vi "GeneralSettings.vi"(11 "notifier":refnum<notifier>) -> ()   [LabVIEW 2013, in "main.lvlib"]
uses:
  main.lvlib
  Controls/Enum Variables.ctl
  Controls/Enum Save Action Events.ctl
  Controls/Enum User Events.ctl
panel:
  out "JournalPositionLabel":string="Journal position i Excel" caption="generalSettingsString"
  in  "CellStr2":string="H49" caption="Højre/Nederst"
  in  "CellStr1":string="A1" caption="Venstre/Øverst"
  in  "LanguageSelectionRing":u16(ring) caption="Sprog" items=["Dansk", "English", "Français"]
  out "generalSettingsString":string
  in  "hyphenationDialogBox":bool caption="Hyphenation"
  # "Ex: A1"
  # "Ex: H49"
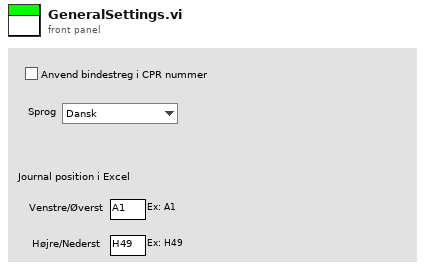
[diagram p1: front panel]
types:
  T1 = typedef "main.lvlib/Enum Variables.ctl" = enum16{"SetAcqFilter", "GetAcqFilter", "Set Filter", "Get Filter", "Set Height", "Get Height", "Set Recorded Height", "Get Recorded Height", "Set Blue Pressure", "Get Blue Pressure", "Set Red Pressure", "Get Red Pressure", "Init", "Reset Pressure", "Set Red Cursors", "Get Red Cursors", "Set Blue Cursors", "Get Blue Cursors", "Set Language", "Get Language", "Set Active Graphs", "Get ActiveGraphs", "Set Method", "Get Method", "Set Encryption", "Get Encryption", "Set ExcelVersion", "Get ExcelVersion", "Set DICOM Avail", "Get DICOM Avail", "Set DICOM Encode", "Get DICOM Encode", "Set JournalExport", "Get JournalExport", "Set Sequence", "Get Sequence", "Set DAQ Connected", "Get DAQ Connected", "Set Current Graph", "Get Current Graph", "Set General Settings", "Get Hyphenation", "Set Arm Calc Method", "Get Arm Calc Method", "Set Dicom Tags", "Get Dicom Tags", "Set BT Serial", "Get BT Serial", "Set BT Accepted Serials", "Get BT Accepted Serials", "Get BT License", "Set BT License"}
  T2 = typedef "main.lvlib/Enum Save Action Events.ctl" = enum16{"LoadReportPath", "SaveReportPath", "Load Graph Path", "Save Graph Path", "LoadDataPath", "SaveDataPath", "Load Template Path", "Save Template Path", "Load PressureFactor", "Save PressureFactor", "Init", "Load Listbox", "Save Listbox", "LoadHospInfo", "SaveHospInfo", "Load DICOM Activation", "Save DICOM Activation", "LoadDICOMInfoWL", "SaveDICOMInfoWL", "LoadDICOMInfoPACS", "SaveDICOMInfoPACS", "Load ArmCalcMethod", "Save ArmCalcMethod", "LoadItemTags", "SaveItemTags", "LoadDICOMEncoding", "SaveDICOMEncoding", "LoadJournalType", "SaveJournalType", "LoadAcqFilterType", "SaveAcqFilterType", "Load Sequence", "Save Sequence", "Load Acquisition Mode", "Save Acquisition Mode", "Load General Settings", "Save General Settings", "Load Language", "Save Language", "Load Dicom Tags", "Save Dicom Tags", "Load BT Serial", "Save BT Serial", "Load BT License", "Save BT License"}
  T3 = typedef "main.lvlib/Enum User Events.ctl" = enum16{"User Event", "Init"}
  T4 = cluster{"hyphenationDialogBox":bool, "LanguageSelectionRing":u16, "CellStr1":string, "CellStr2":string}
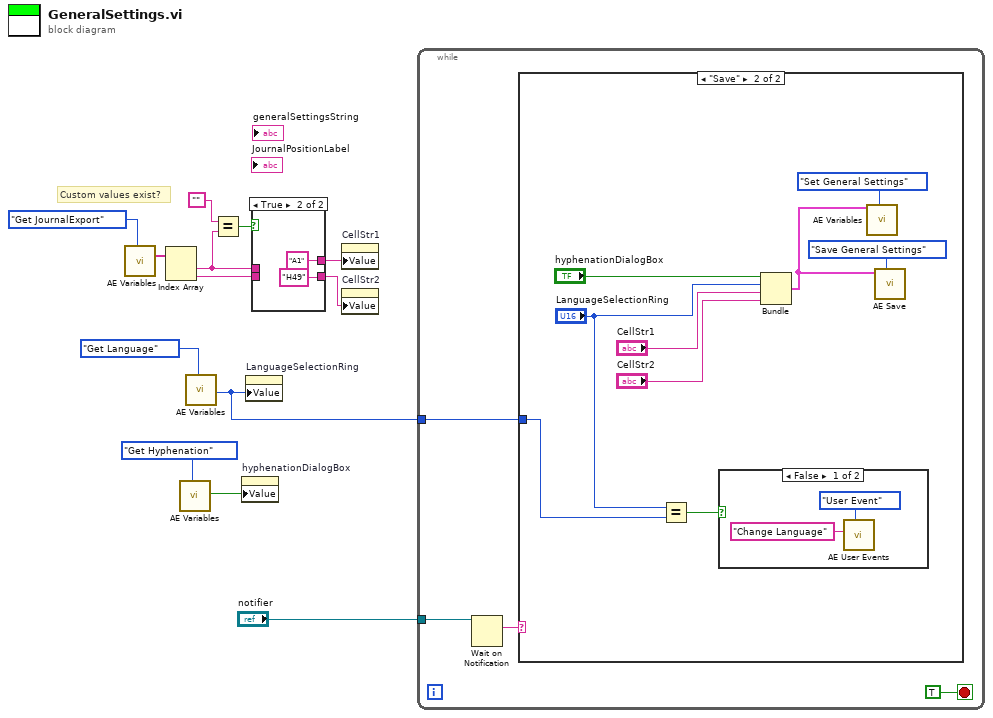
[diagram p0: block diagram]
diagram:
  # "Custom values exist?"
  n1 = call "AE Variables.vi"("Action"=Enum_Variables."Get JournalExport") -> ("stringArray"=w7:string[])  [unwired: 11 in, 7 out]
  n2 = Index Array(array=w7) -> (element #1=w4:string, element #2=w3:string)  [unwired: 2 in]
  n3 = call "AE Variables.vi"("Action"=Enum_Variables."Get Hyphenation") -> ("BooleanOut"=w11:bool)  [unwired: 11 in, 7 out]
  n4 = call "AE Variables.vi"("Action"=Enum_Variables."Get Language") -> ("RingOut"=w9:u16)  [unwired: 11 in, 7 out]
  n5 = Equal?(x="", y=w4) -> (x = y?=w5:bool)
  n6 = property on="hyphenationDialogBox" class="Bool (strict)"("Value"=w11) -> ()  [unwired: 2 in, 2 out]
  n7 = property on="LanguageSelectionRing" class="Ring (strict)"("Value"=w9) -> ()  [unwired: 2 in, 2 out]
  n8 = case shown="True" w5 {
    tunnel: w4 -> [w15 _]
    tunnel: w3 -> [w14 _]
    tunnel: [w15 "A1"] -> w2
    tunnel: [w14 "H49"] -> w1
    frame False {
    }
    frame True {
    }
  }
  n9 = property on="CellStr1" class="Str"("Value"=w2) -> ()  [unwired: 2 in, 2 out]
  n10 = property on="CellStr2" class="Str"("Value"=w1) -> ()  [unwired: 2 in, 2 out]
  n11 = while {
    tunnel: "notifier" -> [w20]
    tunnel: w9 -> [w18]
    stop <- TRUE stop-if-true
    n12 = Wait on Notification(notifier=w20) -> (notification=w21:string)  [unwired: 3 in, 3 out]
    n13 = case shown="\"Save\"" w21 {
      tunnel: w18 -> [_ w26]
      frame "Cancel", Default {
      }
      frame "Save" {
        n14 = Equal?(x="LanguageSelectionRing", y=w26) -> (x = y?=w25:bool)
        n15 = case shown="False" w25 {
          frame False {
            n16 = call "AE User Events.vi"("Action"=Enum_User_Events."User Event", "User Event"="Change Language") -> ()  [unwired: 8 in, 2 out]
          }
          frame True {
          }
        }
        n17 = Bundle("hyphenationDialogBox"="hyphenationDialogBox", "LanguageSelectionRing"="LanguageSelectionRing", "CellStr1"="CellStr1", "CellStr2"="CellStr2") -> (w24:T4)  [unwired: 1 in]
        n18 = call "AE Variables.vi"("VariantIn"=w24, "Action"=Enum_Variables."Set General Settings") -> ()  [unwired: 10 in, 8 out]
        n19 = call "AE Save.vi"("Variant In"=w24, "Action"=Enum_Save_Action_Events."Save General Settings") -> ()  [unwired: 7 in, 2 out]
      }
    }
  }
